vi "Bundle Script_Property Insert.vi"(6 "Dialog Choice":enum32{"Choice 1", "Choice 2"}(radio), 8 "error in":errorcluster, 9 "Property Array":T2(array[cluster]), 11 "Affected Items":T1) -> (0 "error out":errorcluster, 2 "Objects":refnum<vi>[](array[refnum]))   [LabVIEW 2023]
uses:
  top/BundleMagic.ctl
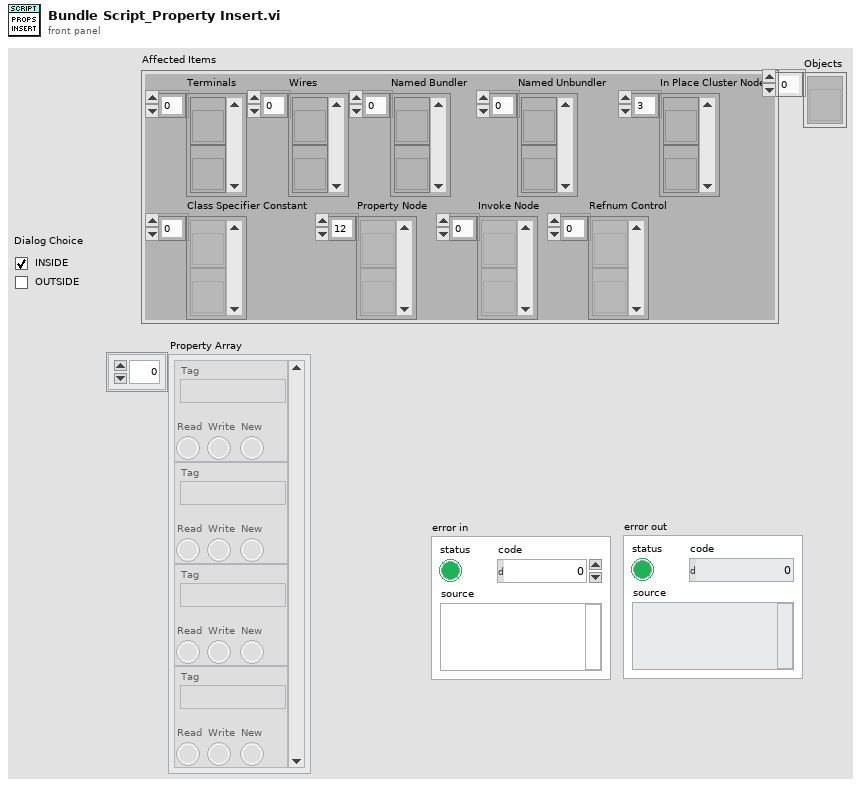
[diagram p1: front panel]
types:
  T1 = typedef "BundleMagic.ctl" = cluster{"Terminals":refnum<vi>[], "Wires":refnum<vi>[], "Named Bundler":refnum<vi>[], "Named Unbundler":refnum<vi>[], "In Place Cluster Node":refnum<vi>[], "Class Specifier Constant":refnum<vi>[], "Property Node":refnum<vi>[], "Invoke Node":refnum<vi>[], "Refnum Control":refnum<vi>[]}
  T2 = cluster{"Tag":string, "Read":bool, "Write":bool, "New":bool}[]
  T3 = cluster{"Index":u16, "Property Type":enum16{"Unknown", "Base", "Scripting", "Private", "Deprecated", "None", "Divider"}, "ID String":string, "Dotted ID String":string, "Class":string, "Parent":string, "Display name full":string, "Display name short":string, "Parents Array":string[], "Indent":u16}
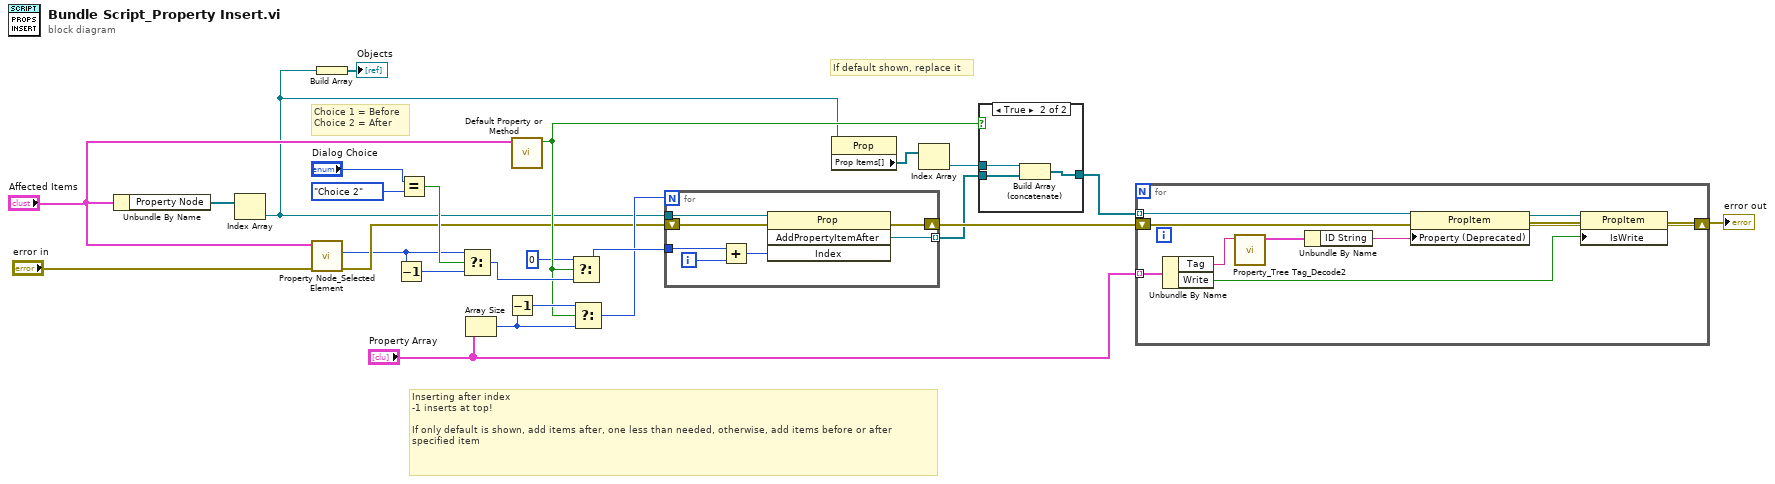
[diagram p0: block diagram]
diagram:
  # "If default shown, replace it"
  # "Inserting after index \n-1 inserts at top!\n\nIf only default is shown, add items after, one less than needed, otherwise, add items before or after specified item"
  # "Choice 1 = Before\nChoice 2 = After"
  n1 = Unbundle By Name("Affected Items") -> ("Property Node"=w24:refnum<vi>[])
  n2 = Index Array(array=w24) -> (element=w2:refnum<vi>)  [unwired: 1 in]
  n3 = call "Property Node_Selected Element.vi"("error in (no error)"="error in", "Affected Items"="Affected Items") -> ("error out"=w4:errorcluster, "index of element"=w1:i32)  [unwired: 4 in, 4 out]
  n4 = Build Array(w2) -> (→"Objects":refnum<vi>[])
  n5 = Decrement(x=w1) -> (x-1=w19:i32)
  n6 = Equal?(x="Dialog Choice", y=enum32{"Choice 1", "Choice 2"}."Choice 2" ("Dialog Choice")) -> (x = y?=w20:bool)
  n7 = Select(t=w1, s=w20, f=w19) -> (s? t:f=w18:i32)
  n8 = Array Size(array="Property Array") -> (size(s)=w10:i32)
  n9 = Decrement(x=w10) -> (x-1=w11:i32)
  n10 = call "Default Property or Method.vi"("Affected Items"="Affected Items") -> ("One default element"=w9:bool)  [unwired: 9 in, 1 out]
  n11 = Select(t=0, s=w9, f=w18) -> (s? t:f=w7:i32)
  n12 = Select(t=w11, s=w9, f=w10) -> (s? t:f=w6:i32)
  n13 = for {
    N: w6 -> [_]
    shift-right: [w26] -> w17
    shift-left: w4 -> [w31]
    tunnel: w2 -> [w30]
    tunnel: w7 -> [w28]
    tunnel: [w25] -> w13 mode=indexing
    i -> [w27]
    n14 = Add(x=w28, y=w27) -> (x+y=w29:i32)
    n15 = invoke class="Prop" method="AddPropertyItemAfter"(reference=w30, error in=w31, "Index"=w29) -> (error out=w26:errorcluster, "AddPropertyItemBefore"=w25:refnum<vi>)  [unwired: 1 in, 2 out]
  }
  "error out" <- w17
  n16 = property class="Prop"(reference=w2) -> ("Prop Items[]"=w15:refnum<vi>[])  [unwired: 1 in, 2 out]
  n17 = Index Array(array=w15) -> (element=w14:refnum<vi>)  [unwired: 1 in]
  n18 = case shown="True" w9 {
    tunnel: w14 -> [_ w35]
    tunnel: w13 -> [w32 w34]
    tunnel: [w32 w33] -> w12
    frame False {
    }
    frame True {
      n19 = Build Array (concatenate)(w35, w34) -> (w33:refnum<vi>[])
    }
  }
  n20 = for {
    shift-right: [w43] -> _
    shift-left: w17 -> [w39]
    tunnel: "Property Array" -> [w45] mode=indexing
    tunnel: w12 -> [w40] mode=indexing
    n21 = Unbundle By Name(w45) -> ("Tag"=w41:string, "Write"=w44:bool)
    n22 = call "Property_Tree Tag_Decode2.vi"("Tag In"=w41) -> ("TagData"=w42:T3)  [unwired: 10 in]
    n23 = Unbundle By Name(w42) -> ("ID String"=w38:string)
    n24 = property class="PropItem"(reference=w40, error in=w39, "Property (Deprecated)"=w38) -> (reference out=w36:refnum<vi>, error out=w37:errorcluster)
    n25 = property class="PropItem"(reference=w36, error in=w37, "IsWrite"=w44) -> (error out=w43:errorcluster)  [unwired: 1 out]
  }
